vi "ShowTexturedPointCloud.vi"(2 "error in (no error)":errorcluster, 3 "TexturedPointCloud Reference in":refnum<k24>) -> (0 "SceneObject out":refnum<vi>, 1 "error out":errorcluster)   [LabVIEW 2023]
uses:
  C:/Mech-Mind/Mech-Eye SDK-2.5.0-c1-dev-01-17/API/dll/net48/MechEyeApiNet.dll
  dll/net48/MechEyeApiNet.dll
  <vilib>/picture/3D Picture Control/Object/Create Object (name).vi
  <vilib>/picture/3D Picture Control/NI_3D Picture Control.lvlib
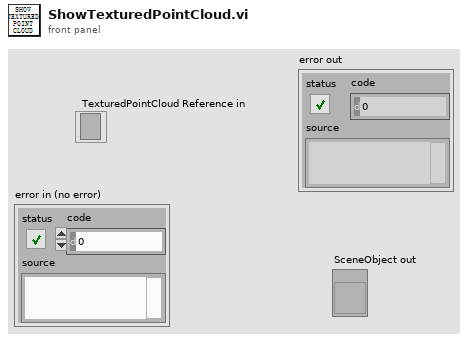
[diagram p1: front panel]
types:
  T1 = enum16{"Overall", "Per Primitive", "Per Vertex", "Binding Off"}
  T2 = enum16{"Points", "Lines", "Line Strip", "Line Loop", "Triangles", "Triangle Strip", "Triangle Fan", "Quads", "Quad Strip", "Polygon"}
  T3 = cluster{"ColorArray[0]":dbl, "ColorArray[1]":dbl, "ColorArray[2]":dbl, "ColorArray[3]":dbl}
  T4 = cluster{"VertArray[0]":sgl, "VertArray[1]":sgl, "VertArray[2]":sgl}
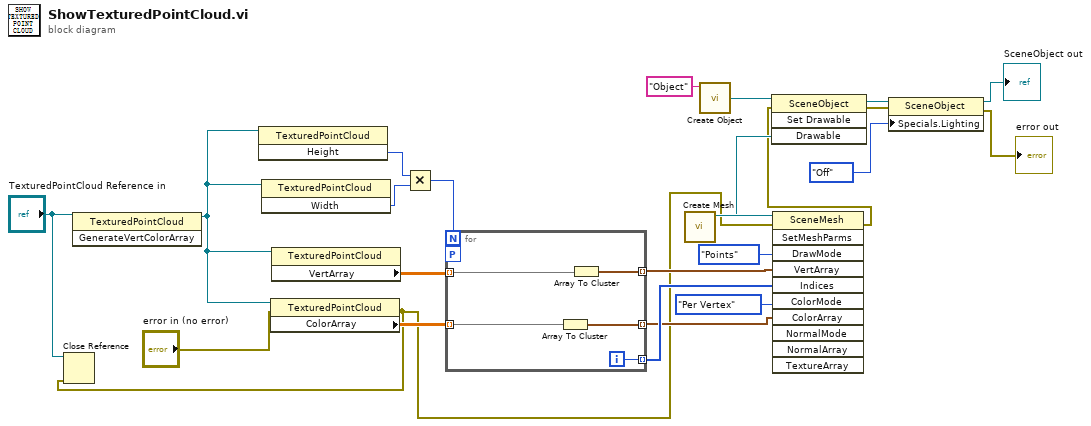
[diagram p0: block diagram]
diagram:
  n1 = invoke class="TexturedPointCloud" method="GenerateVertColorArray"(reference="TexturedPointCloud Reference in") -> (reference out=w4:refnum<k24>)  [unwired: 2 in, 2 out]
  n2 = invoke class="TexturedPointCloud" method="Height"(reference=w4) -> ("Height"=w21:u64)  [unwired: 2 in, 2 out]
  n3 = invoke class="TexturedPointCloud" method="Width"(reference=w4) -> ("Width"=w23:u64)  [unwired: 2 in, 2 out]
  n4 = property class="TexturedPointCloud"(reference=w4, error in="error in (no error)") -> (error out=w2:errorcluster, "ColorArray"=w5:dbl[][])  [unwired: 1 out]
  n5 = Close Reference(reference="TexturedPointCloud Reference in", error in (no error)=w2) -> ()  [unwired: 1 out]
  n6 = property class="TexturedPointCloud"(reference=w4) -> ("VertArray"=w6:sgl[][])  [unwired: 1 in, 2 out]
  n7 = Multiply(x=w21, y=w23) -> (x*y=w22:u64)
  n8 = for {
    N: w22 -> [_]
    tunnel: [w27] -> w8 mode=indexing
    tunnel: [w29] -> w24 mode=indexing
    tunnel: [w25] -> w7 mode=indexing
    workers-P: _ -> [_]
    tunnel: w6 -> [w28] mode=indexing
    tunnel: w5 -> [w26] mode=indexing
    i -> [w29]
    n9 = Array To Cluster(array=w26) -> (cluster=w25:T3)
    n10 = Array To Cluster(array=w28) -> (cluster=w27:T4)
  }
  n11 = call <vilib>:"Create Mesh.vi"() -> ("New Mesh Refnum"=w14:refnum<vi>)  [unwired: 10 in, 1 out]
  n12 = call-poly <vilib>:"Create Object.vi"("Name"="Object") -> ("Scene:New Object"=w15:refnum<vi>)  [unwired: 9 in, 1 out]
  n13 = invoke class="SceneMesh" method="SetMeshParms"(reference=w14, error in=w2, "DrawMode"=T2."Points" ("Draw Mode"), "VertArray"=w8, "Indices"=w24, "ColorMode"=T1."Per Vertex" ("Color Binding Mode"), "ColorArray"=w7) -> (reference out=w13:refnum<vi>, error out=w9:errorcluster)  [unwired: 4 in, 9 out]
  n14 = invoke class="SceneObject" method="Set Drawable"(reference=w15, error in=w9, "Drawable"=w13) -> (reference out=w12:refnum<vi>, error out=w11:errorcluster)  [unwired: 1 in, 2 out]
  n15 = property class="SceneObject"(reference=w12, error in=w11, "Specials.Lighting"=enum16{"Inherit Value", "Off", "On"}."Off" ("Specials:Lighting")) -> (reference out=→"SceneObject out":refnum<vi>, error out=→"error out":errorcluster)
